vi "Handle Key Event.vi"(8 "error in (no error)":errorcluster, 10 "Key Event Data":T1, 11 "Terminal in":refnum<class "Terminal.lvclass">) -> (0 "error out":errorcluster, 3 "Terminal out":refnum<class "Terminal.lvclass">)   [LabVIEW 2020, in "Terminal.lvlib" / "Terminal.lvclass"]
uses:
  Terminal.lvclass
  Key Event Data.ctl
  <vilib>/event_ctls.llb/eventvkey.ctl
  Terminal.lvclass/Terminal.ctl
  Terminal.lvlib
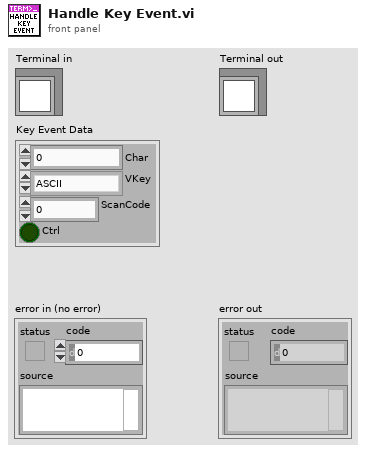
[diagram p1: front panel]
types:
  T1 = typedef "Terminal.lvlib/Key Event Data.ctl" = cluster{"Char":i16, "VKey":T2, "ScanCode":i16, "Ctrl":bool}
  T2 = typedef "eventvkey.ctl" = enum16{"ASCII", "Enter", "Return", "Shift", "Ctrl", "Alt", "Cmd", "Opt", "Caps", "NumLock", "Clear", "Break", "Up", "Down", "Left", "Right", "Insert", "Delete", "Home", "End", "PageUp", "PageDown", "Escape", "Help", "Pause", "ScrollLock", "F1", "F2", "F3", "F4", "F5", "F6", "F7", "F8", "F9", "F10", "F11", "F12", "F13", "F14", "F15", "F16", "F17", "F18", "F19", "F20", "F21", "F22", "F23", "F24", "Play", "VolumeUp", "VolumeDown", "Mute", "Two Byte Char"}
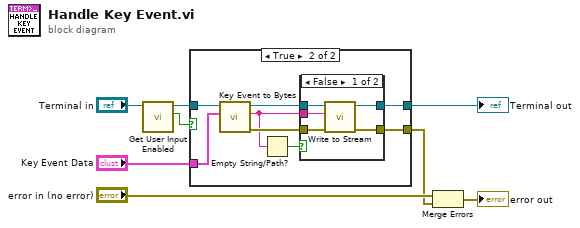
[diagram p0: block diagram]
diagram:
  n1 = call "Get User Input Enabled.vi"("Terminal in"="Terminal in") -> ("User Input Enabled"=w1:bool, "Terminal out"=w2:refnum<class "Terminal.lvclass">)  [unwired: 8 in, 1 out]
  n2 = case shown="True" w1 {
    tunnel: "Key Event Data" -> [_ w17]
    tunnel: [w9 w15] -> w6
    tunnel: [_ w13] -> w4
    tunnel: w2 -> [w9 w10]
    frame False {
    }
    frame True {
      n3 = call "Key Event to Bytes.vi"("Key Event Data"=w17, "Terminal in"=w10) -> ("error out"=w14:errorcluster, "String"=w12:string, "Terminal out"=w16:refnum<class "Terminal.lvclass">)  [unwired: 7 in]
      n4 = Empty String/Path?(string/path=w12) -> (empty?=w11:bool)
      n5 = case shown="False" w11 {
        tunnel: w16 -> [w22 w23]
        tunnel: [w19 w23] -> w15
        tunnel: w14 -> [w21 w24]
        tunnel: [w20 w24] -> w13
        tunnel: w12 -> [w18 _]
        frame False {
          n6 = call "Write to Stream.vi"("error in (no error)"=w21, "Data"=w18, "Terminal in"=w22) -> ("error out"=w20:errorcluster, "Terminal out"=w19:refnum<class "Terminal.lvclass">)  [unwired: 7 in]
        }
        frame True {
        }
      }
    }
  }
  "Terminal out" <- w6
  n7 = Merge Errors("error in (no error)", w4) -> (→"error out":errorcluster)
